vi "Function_Yellow Spot #2.vi"(8 "Error in":errorcluster, 9 "CoordSys In":T2 {"Measurement System"."Axis Reference" items=["Direct", "Indirect"]; "Measurement System"."Angle (deg)" format="%.2f"; "Measurement System"."Origin"."Y" format="%.2f"; "Measurement System"."Origin"."X" format="%.2f"; "Reference System"."Axis Reference" items=["Direct", "Indirect"]; "Reference System"."Angle (deg)" format="%.2f"; "Reference System"."Origin"."Y" format="%.2f"; "Reference System"."Origin"."X" format="%.2f"}, 10 "Data Cluster In":cluster{"Name":string, "Variant In":variant}, 11 "Image Src In":T4) -> (0 "Error out":errorcluster, 2 "ROI Descriptor out":T1 {"Contours"."Type" items=["No Selection", "Point", "Line", "Rectangle", "Oval", "Polygon", "Freehand Region", "Annulus", "Unused2", "Unused3", "Broken Line", "Freehand Line", "Rotated Rectangle"]}, 3 "Objects":T3(array[cluster]) {"Area" format="%.2f"; "Object Center"."Y" format="%.2f"; "Object Center"."X" format="%.2f"})   [LabVIEW 2013]
uses:
  <vilib>/vision/Image Controls.llb/IMAQ Image.ctl
  Control/Control_Yellow Spot.ctl
  <vilib>/vision/NI_Vision_Development_Module.lvlib
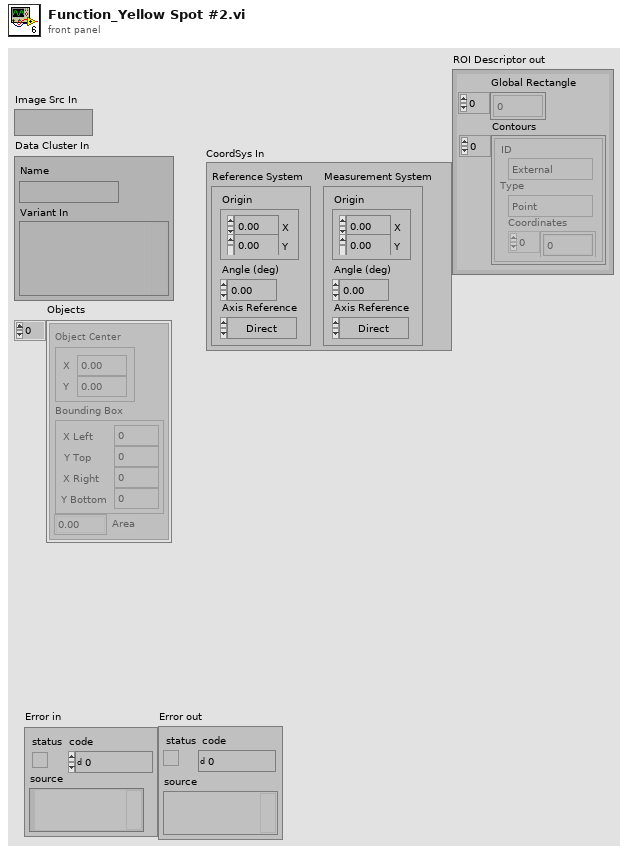
[diagram p1: front panel]
types:
  T1 = typedef "ROI Descriptor" = cluster{"Global Rectangle":i32[], "Contours":cluster{"ID":enum32{"External", "Internal"}, "Type":u32, "Coordinates":i32[]}[]}
  T2 = typedef "IMAQ Coordinate System" = cluster{"Reference System":cluster{"Origin":cluster{"X":sgl, "Y":sgl}, "Angle (deg)":sgl, "Axis Reference":u32}, "Measurement System":cluster{"Origin":cluster{"X":sgl, "Y":sgl}, "Angle (deg)":sgl, "Axis Reference":u32}}
  T3 = cluster{"Object Center":cluster{"X":dbl, "Y":dbl}, "Bounding Box":cluster{"X Left":dbl, "Y Top":dbl, "X Right":dbl, "Y Bottom":dbl}, "Area":dbl}[]
  T4 = typedef "IMAQ Image.ctl" = refnum<image>
  T5 = typedef "Control_Yellow Spot.ctl" = cluster{"Name":string, "ROI":cluster{"Global Rectangle":i32[], "Contours":cluster{"ID":enum32{"External", "Internal"}, "Type":u32, "Coordinates":i32[]}[]}, "Magnification(独闯)":i32, "»Ö­È(¶À´³)":i16, "Settings(独闯)":cluster{"Objects":enum16{"Bright Objects", "Dark Objects"}, "Threshold":i32, "Min Object Size":bool, "Min Size":i32, "Max Object Size":bool, "Max Size":i32}}
  T6 = cluster{"Origin":cluster{"X":sgl, "Y":sgl}, "Angle (deg)":sgl, "Axis Reference":u32}
  T7 = cluster{"Global Rectangle":i32[], "Contours":cluster{"ID":enum32{"External", "Internal"}, "Type":u32, "Coordinates":i32[]}[]}
  T8 = cluster{"Objects":enum16{"Bright Objects", "Dark Objects"}, "Threshold":i32, "Min Object Size":bool, "Min Size":i32, "Max Object Size":bool, "Max Size":i32}
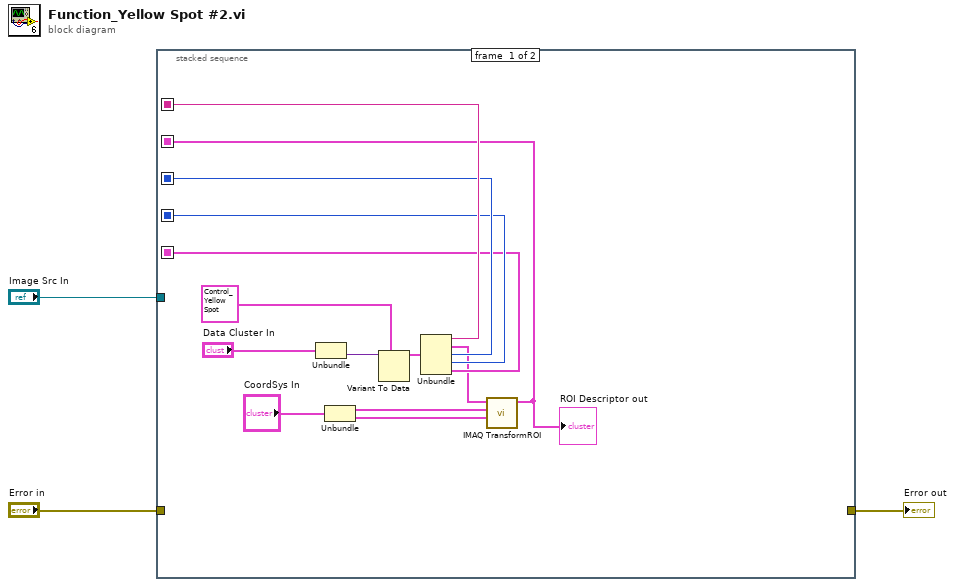
[diagram p0: block diagram]
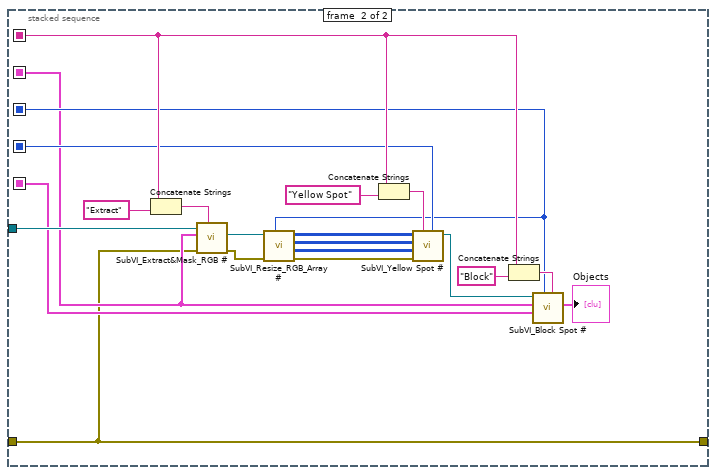
[diagram p2: hidden frame]
diagram:
  n1 = stacked-sequence {
    seq-local: [w12 _] -> [_ w23]
    seq-local: [w4 _] -> [_ w20]
    seq-local: [w11 _] -> [_ w21]
    seq-local: [w10 _] -> [_ w22]
    seq-local: [w9 _] -> [_ w19]
    tunnel: "Error in" -> [_ w18]
    tunnel: [_ w18] -> w2
    tunnel: "Image Src In" -> [_ w30]
    frame #0 {
      n2 = Unbundle("Data Cluster In") -> ("Variant In"=w14:variant)  [unwired: 1 out]
      n3 = Unbundle("CoordSys In") -> ("Reference System"=w7:T6, "Measurement System"=w6:T6)
      n4 = Variant To Data(type=T5 {"Name"="", "ROI"={"Global Rectangle"=[], "Contours"=[]}, "Magnification(独闯)"=0, "»Ö­È(¶À´³)"=40, "Settings(独闯)"={"Objects"=enum."Bright Objects", "Threshold"=128, "Min Object Size"=FALSE, "Min Size"=3, "Max Object Size"=FALSE, "Max Size"=100}} ("独闯_Setting"), Variant=w14) -> (data=w13:T5)  [unwired: 1 in, 1 out]
      n5 = Unbundle(w13) -> ("Name"=w12:string, "ROI"=w5:T7, "Magnification(独闯)"=w11:i32, "»Ö­È(¶À´³)"=w10:i16, "Settings(独闯)"=w9:T8)
      n6 = call "IMAQ TransformROI"("New Reference"=w6, "Base Reference"=w7, "ROI Descriptor"=w5) -> ("ROI Descriptor out"=w4:T1)  [unwired: 7 in, 1 out]
      "ROI Descriptor out" <- w4
    }
    frame #1 {
      n7 = Concatenate Strings(w23, "Extract" ("Image Register Name")) -> (w28:string)
      n8 = call "SubVI_Extract&Mask_RGB #.vi"("Image Register Name"=w28, "Error in"=w18, "ROI Descriptor"=w20, "Image Src In"=w30) -> ("Error out"=w33:errorcluster, "Image Dst Out"=w37:T4)  [unwired: 4 in, 2 out]
      n9 = call "SubVI_Resize_RGB_Array #.vi"("Magnification"=w21, "Error In"=w33, "Image In"=w37) -> ("Error Out"=w32:errorcluster, "B"=w36:u8[][], "G"=w35:u8[][], "R"=w31:u8[][])  [unwired: 5 in]
      n10 = Concatenate Strings(w23, "Yellow Spot" ("Image Register Name")) -> (w27:string)
      n11 = call "SubVI_Yellow Spot #.vi"("»Ö­È"=w22, "Image Register Name"=w27, "Error In"=w32, "B"=w36, "G"=w35, "R"=w31) -> ("Image Out"=w34:T4)  [unwired: 4 in, 1 out]
      n12 = Concatenate Strings(w23, "Block" ("Image Register Name")) -> (w25:string)
      n13 = call "SubVI_Block Spot #.vi"("Image Register Name"=w25, "Magnification"=w21, "Settings"=w19, "ROI Descriptor"=w20, "Image In"=w34) -> ("Objects"=→"Objects":T3)  [unwired: 5 in, 1 out]
    }
  }
  "Error out" <- w2
